vi "Log.vi"(7 "severity":T1, 10 "data (none)":variant, 11 "message":string) -> ()   [LabVIEW 2018, in "GLog.lvlib"]
uses:
  GLog.lvlib
  Log Levels.ctl
  registry/Registry.lvlib
panel:
  # "Locals"
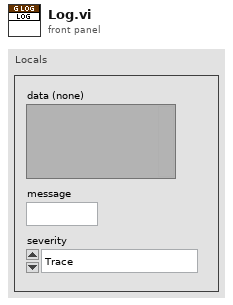
[diagram p1: front panel]
types:
  T1 = typedef "GLog.lvlib/Log Levels.ctl" = enum16{"Trace", "Debug", "Info", "Warning", "Error", "Critical"}
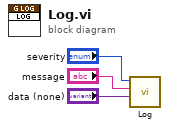
[diagram p0: block diagram]
diagram:
  n1 = call "Log.vi"("data"="data (none)", "message"="message", "level"="severity") -> ()  [unwired: 9 in]
